vi "DataViewer.vi"() -> ()   [LabVIEW 2025]
uses:
  Controls/Dependand_Variables.ctl
  Controls/State.ctl
  <vilib>/Utility/miscctls.llb/LVRowAndColumnUnsignedTypeDef.ctl
panel:
  in  "Btt:Down":bool
  in  "Btt:Up":bool
  out "2D":T1
  out "Horizontal":T1
  out "Vertical":T1
  out "Duration [min]":dbl
  out "End":timestamp
  out "Begin":timestamp
  in  "Stop":bool
  out "Raw Data":i32(listbox)
  in  "Combo Box":string(combo)
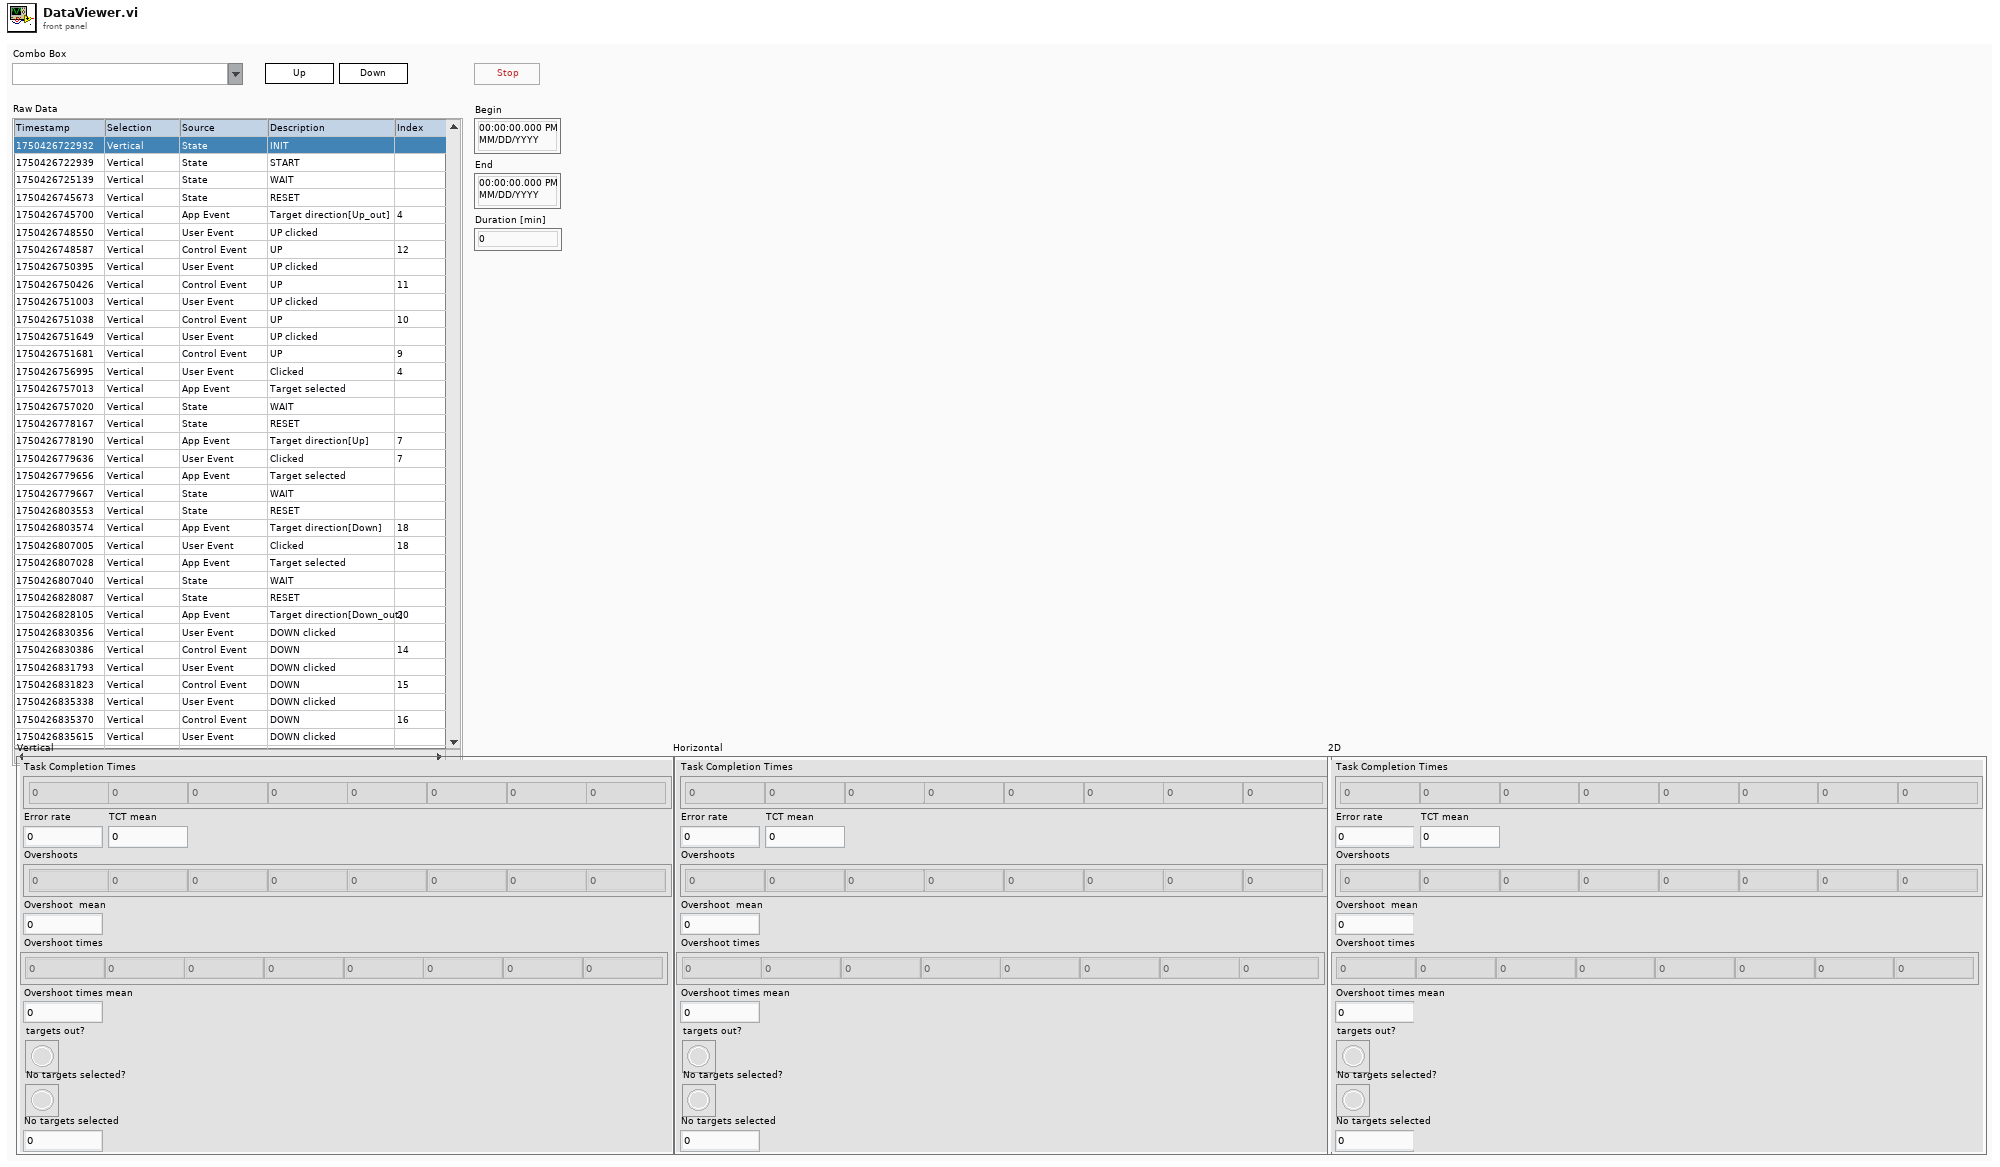
[diagram p1: front panel]
types:
  T1 = typedef "Dependand_Variables.ctl" = cluster{"Task Completion Times":dbl[], "TCT mean":dbl, "Error rate":i32, "Overshoots":i32[], "Overshoot  mean":dbl, "Overshoot times":dbl[], "Overshoot times mean":dbl, "targets out?":bool[], "No targets selected?":bool[], "No targets selected":i32}
  T2 = typedef "State.ctl" = enum16{"Init", "Idle", "Analyze", "End"}
  T3 = typedef "LVRowAndColumnUnsignedTypeDef.ctl" = cluster{"Row":u32, "Column":u32}
  T4 = typedef "LVComboBoxStrsAndValuesArrayTypeDef.ctl" = cluster{"String":string, "Value":string}[]
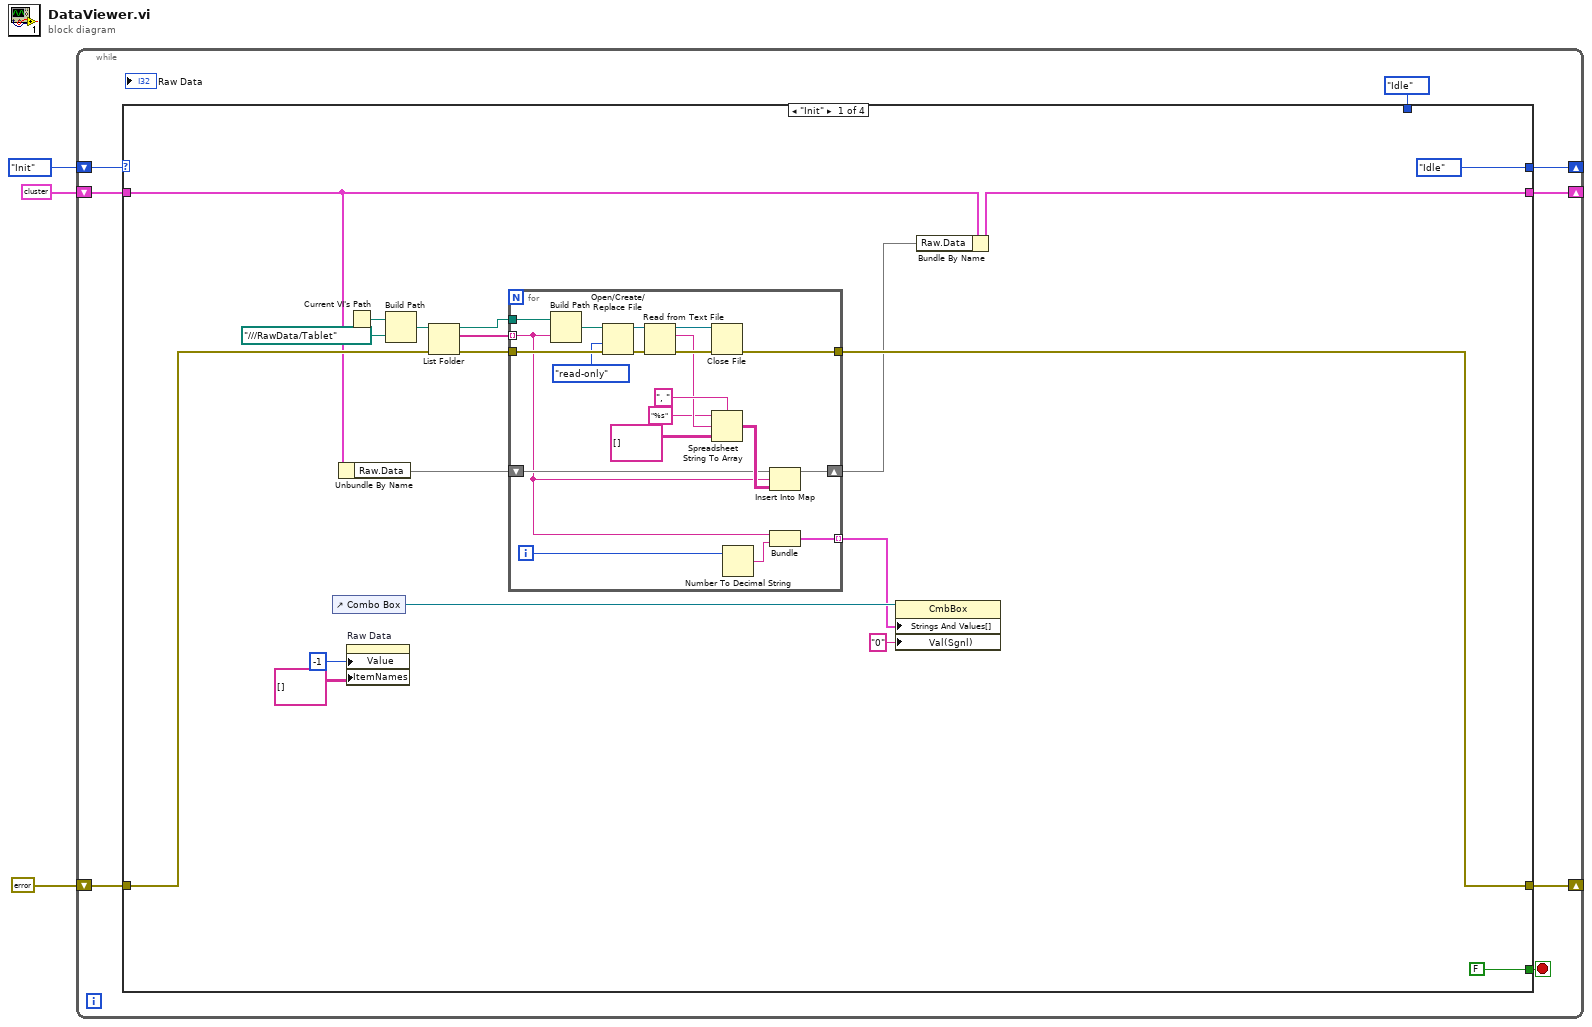
[diagram p0: block diagram]
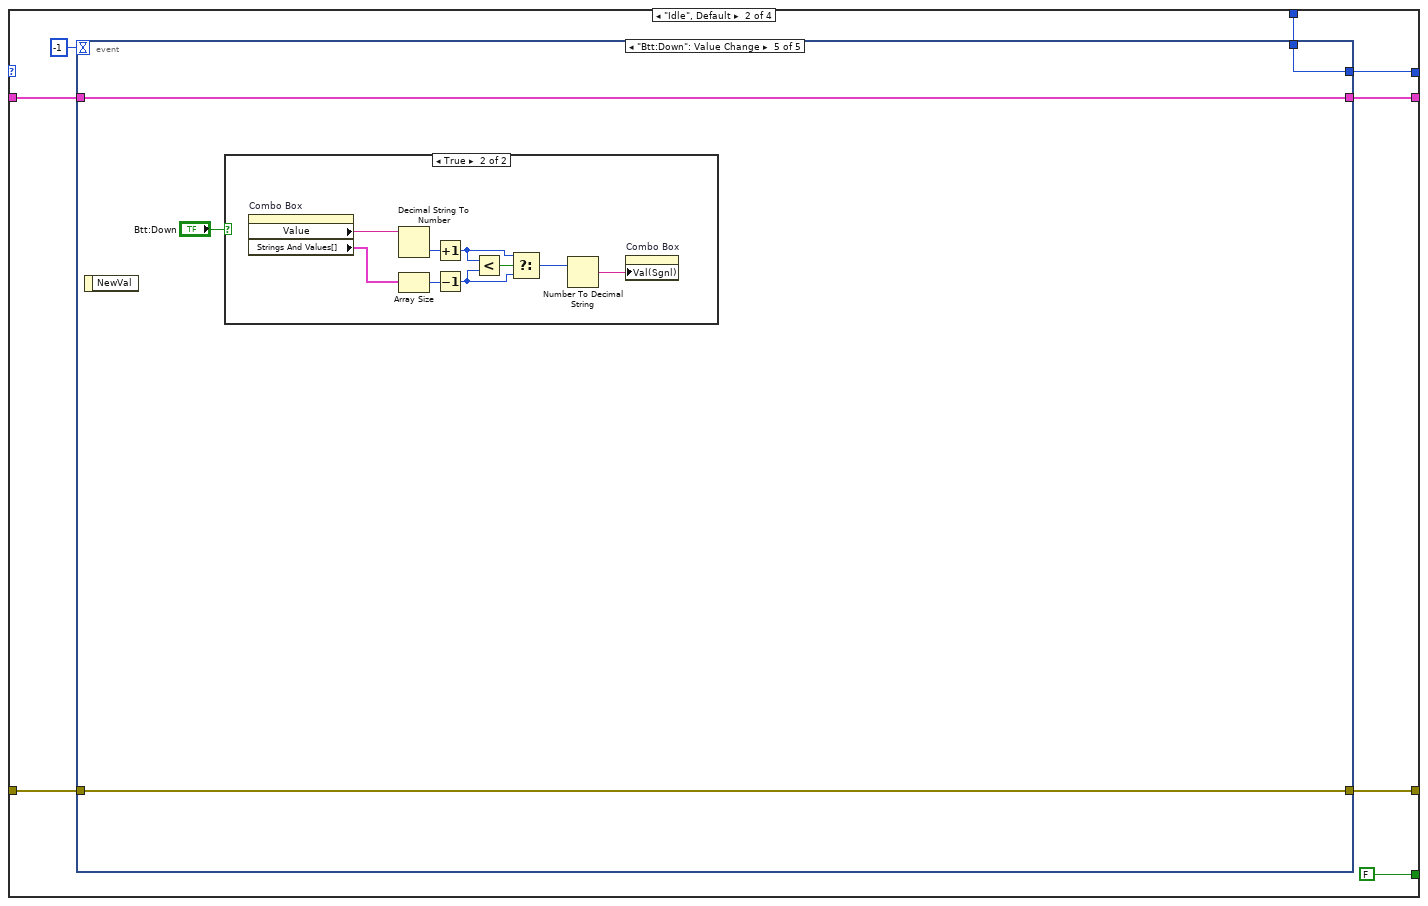
[diagram p2: hidden frame]
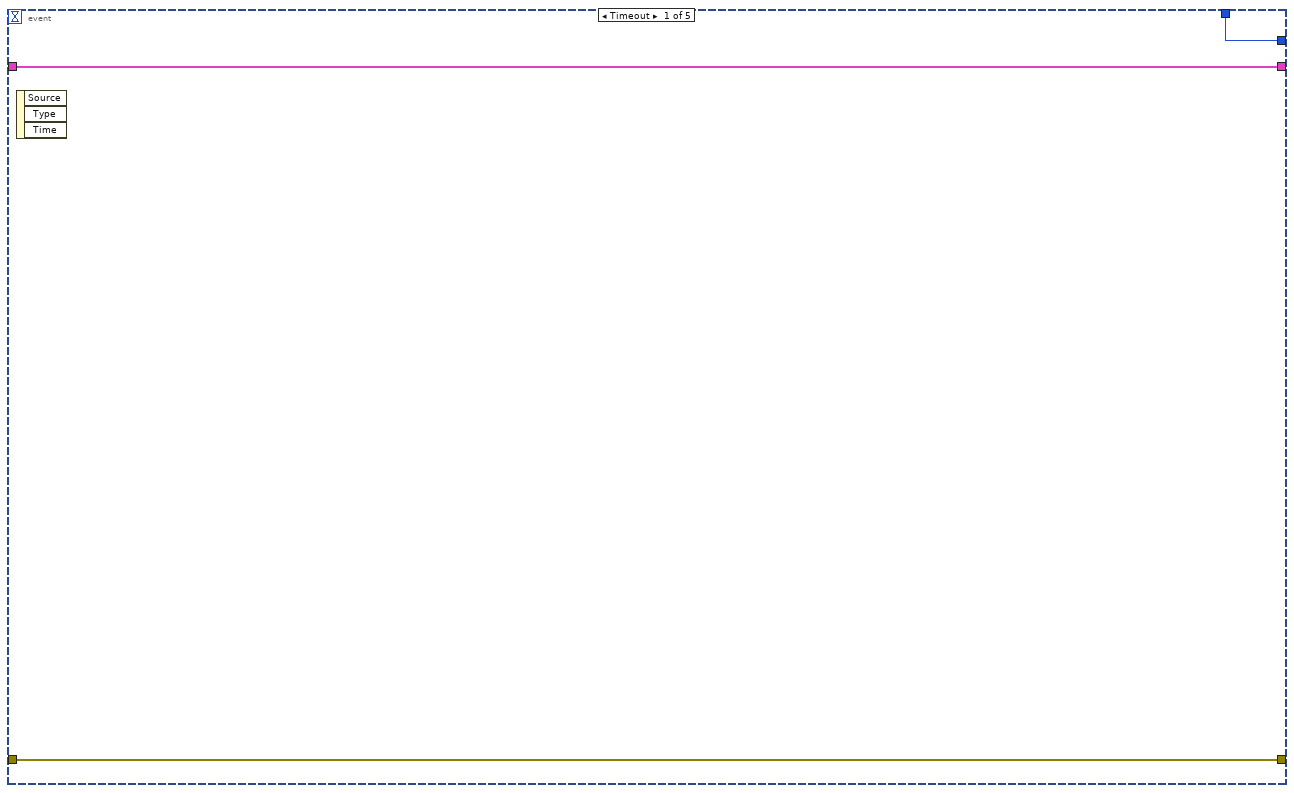
[diagram p3: hidden frame]
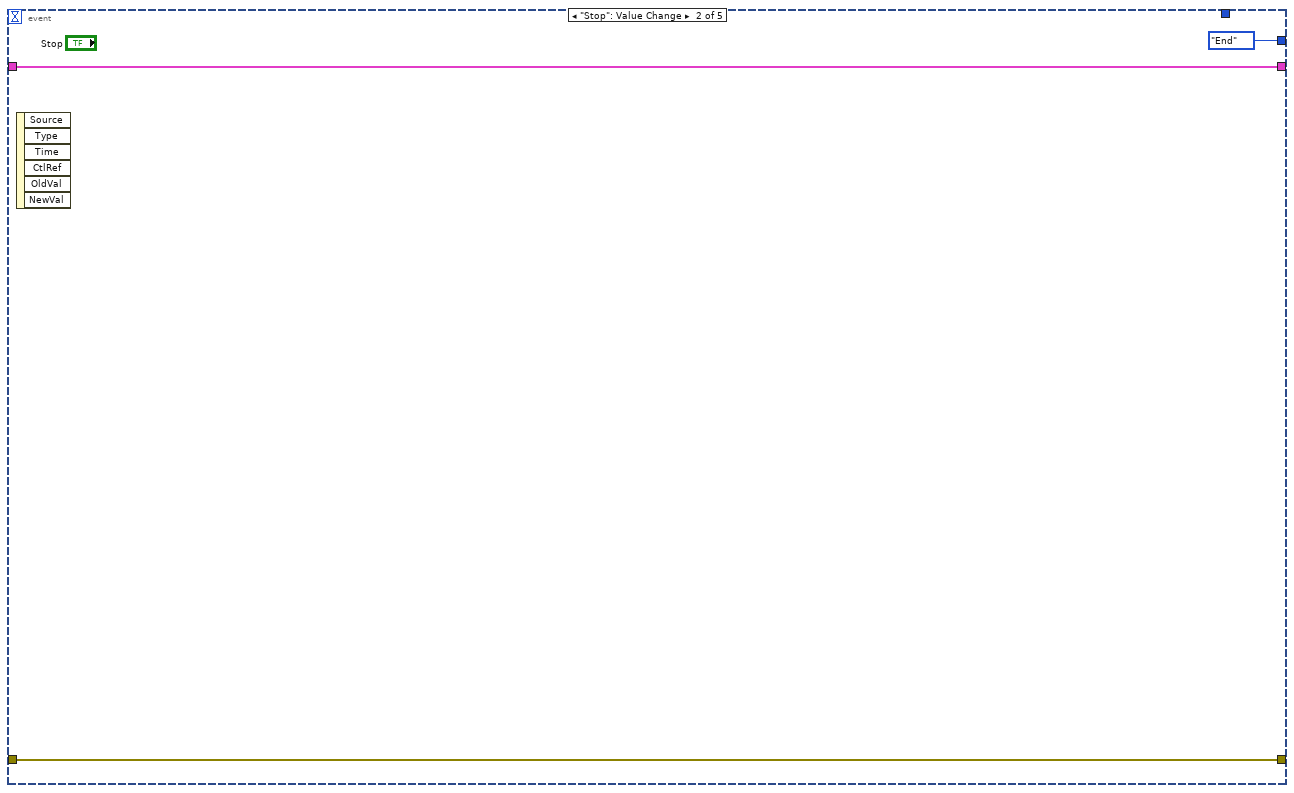
[diagram p4: hidden frame]
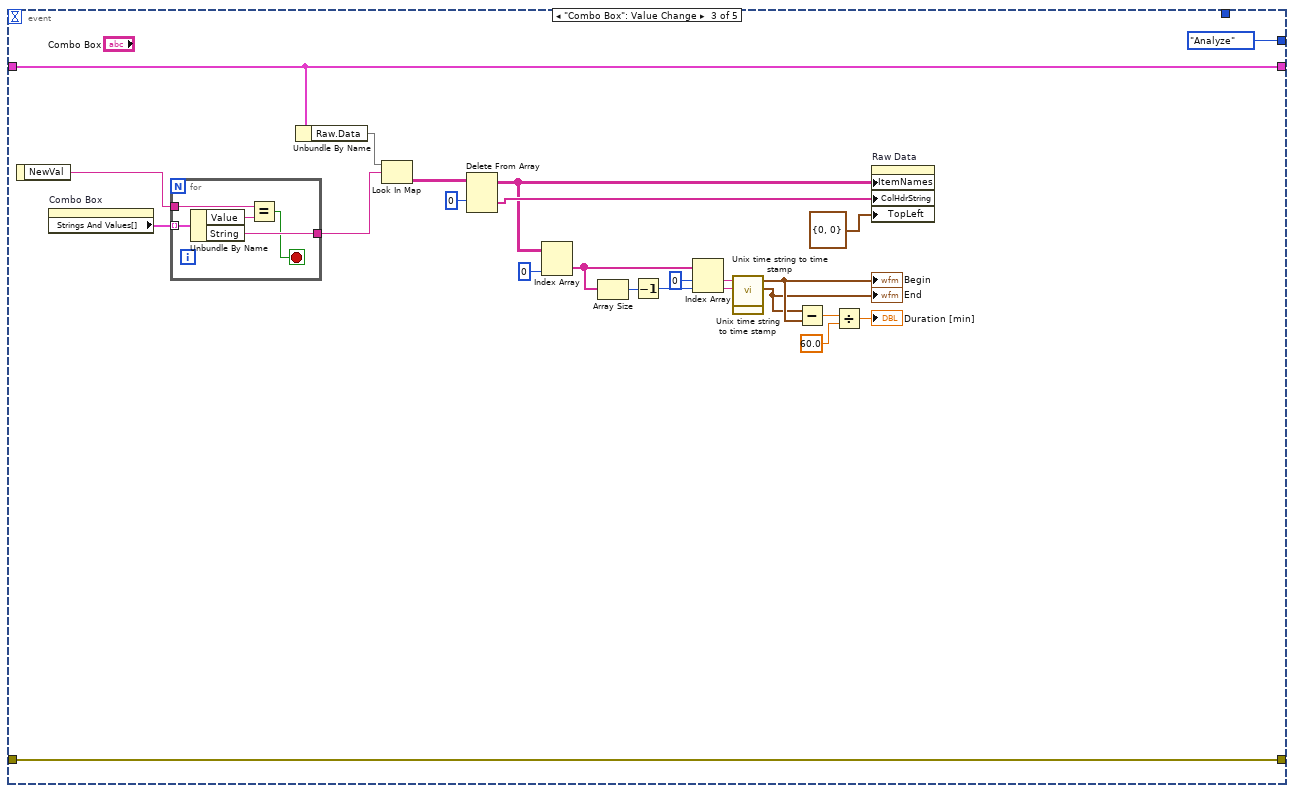
[diagram p5: hidden frame]
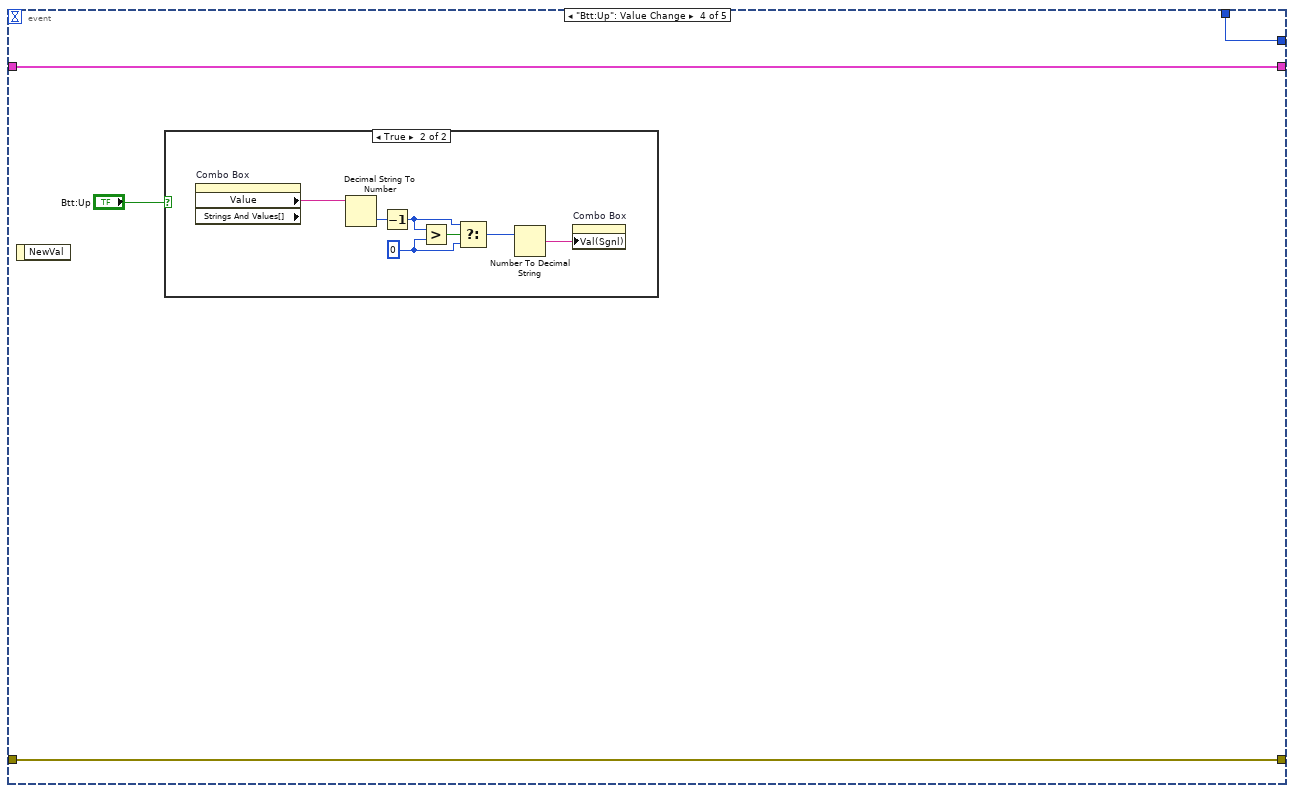
[diagram p6: hidden frame]
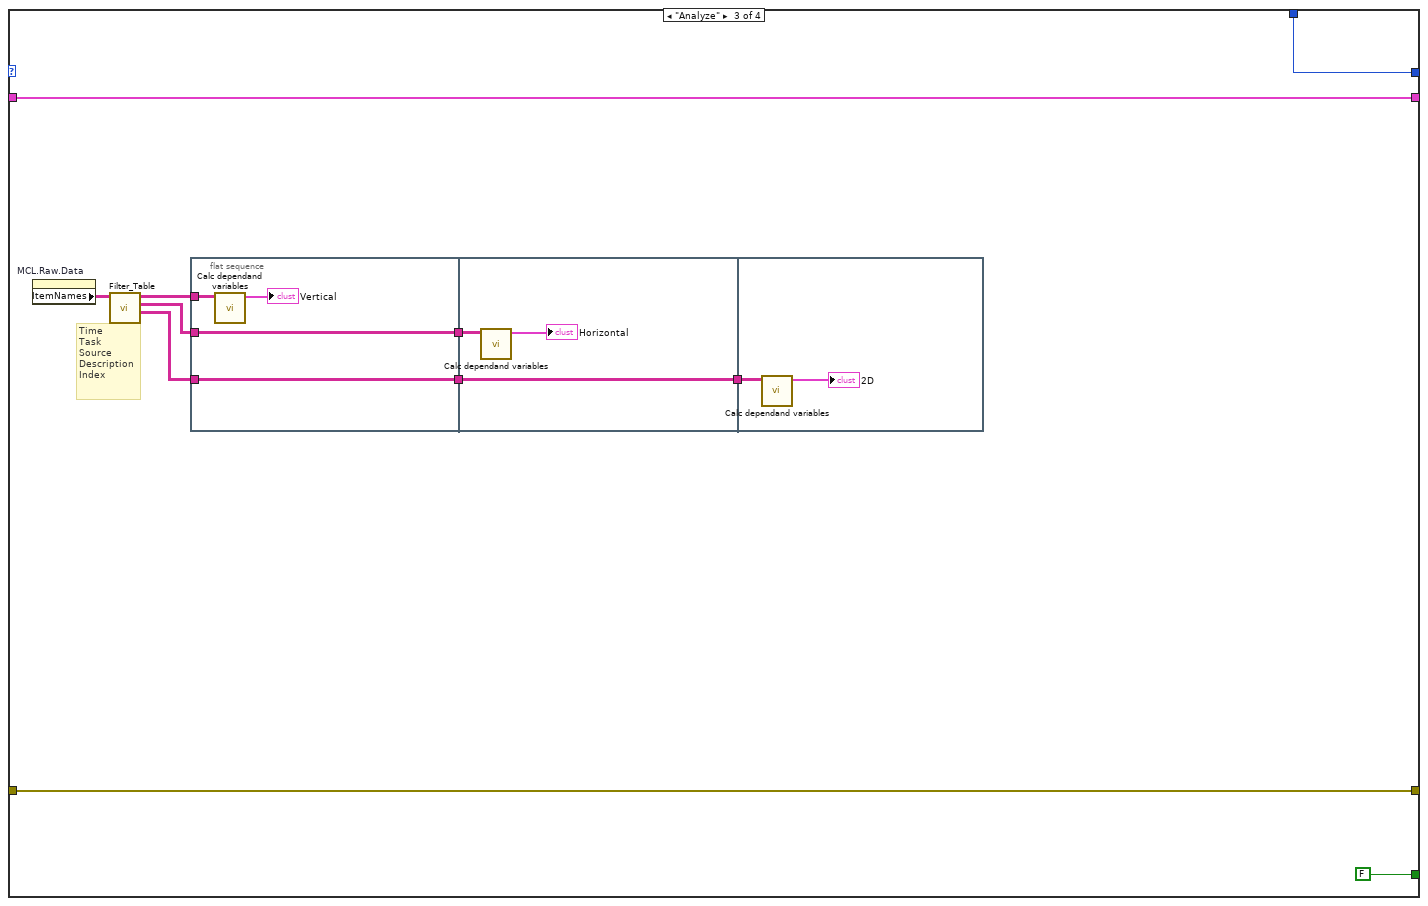
[diagram p9: hidden frame]
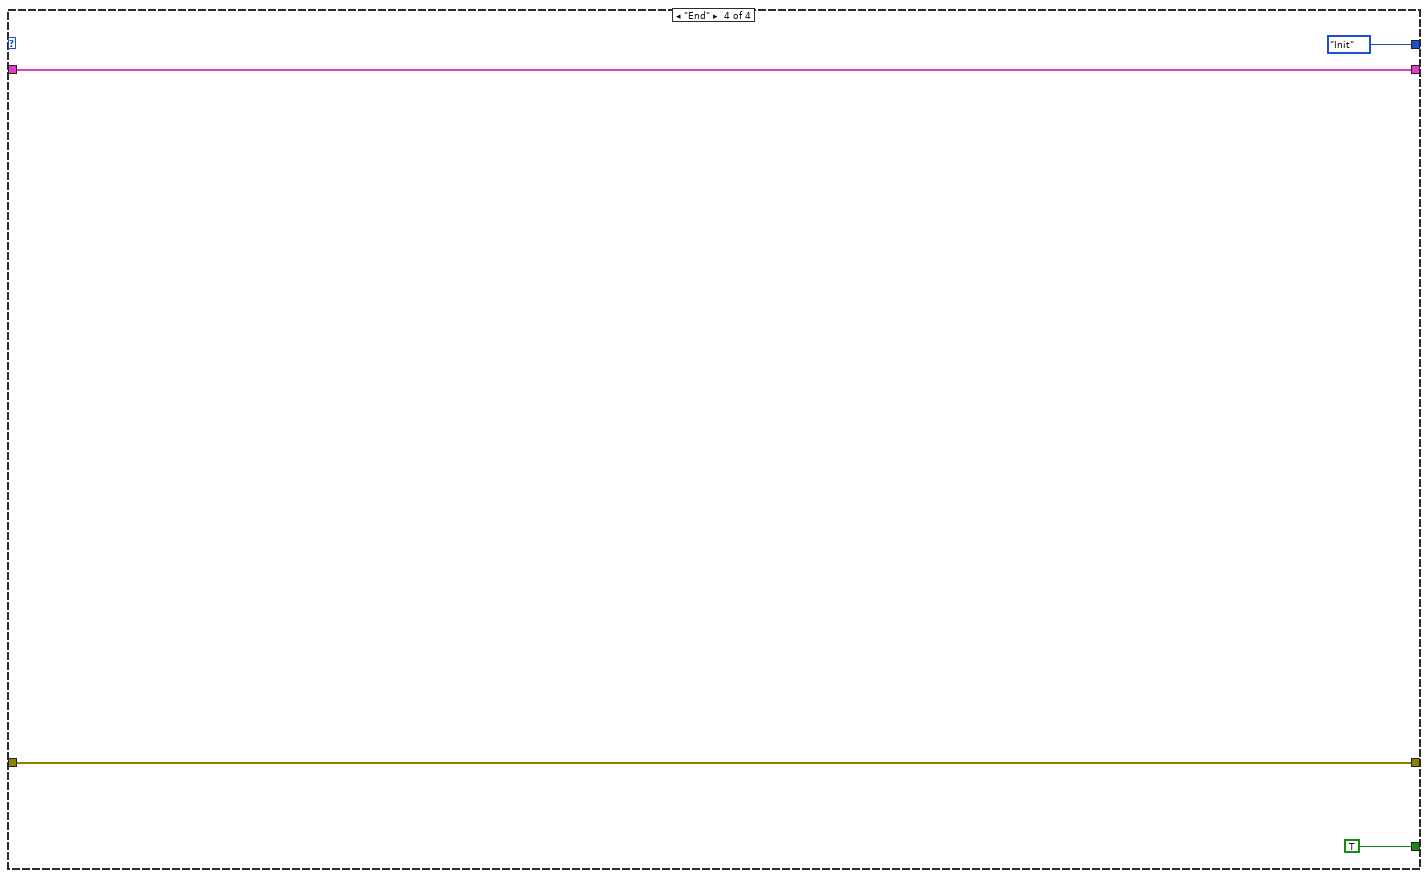
[diagram p10: hidden frame]
diagram:
  n1 = while {
    shift-right: [w9] -> _
    shift-left: errorcluster {"status"=FALSE, "code"=0, "source"=""} ("error constant") -> [w10]
    shift-right: [w8] -> _
    shift-left: State."Init" -> [w11]
    shift-right: [w5] -> _
    shift-left: cluster{"Raw.Data":map{string, string[][]}} {"Raw.Data"={}} -> [w6]
    stop <- w4 stop-if-true
    n2 = case shown="\"Init\"" w11 {
      tunnel: w10 -> [w26 w57 w126 w141]
      tunnel: [w25 w58 w126 w141] -> w9
      tunnel: [State."Idle" w55 w128 State."Init"] -> w8
      tunnel: State."Idle" -> [_ w54 w128 _]
      tunnel: w6 -> [w22 w52 w127 w138]
      tunnel: [w23 w53 w127 w138] -> w5
      tunnel: [FALSE FALSE FALSE TRUE] -> w4
      frame "Init" {
        n3 = control-ref of="Combo Box"() -> (w29:refnum<vi>)
        n4 = Unbundle By Name(w22) -> ("Raw.Data"=w21:map{string, string[][]})
        n5 = Current VI's Path() -> (path=w14:path)
        n6 = property on="Raw Data" class="MCListbox (strict)"("Value"=-1 ("Multicolumn Listbox"), "ItemNames"=string[][] [] ("Item Names")) -> ()  [unwired: 2 in, 2 out]
        n7 = Build Path(base path=w14, name or relative path=path "../../../RawData/Tablet") -> (appended path=w12:path)
        n8 = List Folder(path=w12, error in=w26) -> (path out=w28:path, filenames=w30:string[], error out=w27:errorcluster)  [unwired: 2 in, 1 out]
        n9 = for {
          tunnel: w27 -> [w50]
          tunnel: w28 -> [w45]
          tunnel: w30 -> [w32] mode=indexing
          tunnel: [w38] -> w25
          shift-right: [w35] -> w20
          shift-left: w21 -> [w36]
          tunnel: [w31] -> w16 mode=indexing
          i -> [w34]
          n10 = Build Path(base path=w45, name or relative path=w32) -> (appended path=w44:path)
          n11 = Open/Create/Replace File(file path (use dialog)=w44, error in=w50, access (0:read/write)=enum16{"read/write", "read-only", "write-only"}."read-only") -> (refnum out=w49:refnum<file>, error out=w48:errorcluster)  [unwired: 3 in, 1 out]
          n12 = Read from Text File(file (use dialog)=w49, error in=w48) -> (refnum out=w47:refnum<file>, text=w41:string, error out=w46:errorcluster)  [unwired: 2 in, 1 out]
          n13 = Close File(refnum=w47, error in=w46) -> (error out=w38:errorcluster)  [unwired: 1 out]
          n14 = Spreadsheet String To Array(delimiter (Tab)=", ", format string="%s", spreadsheet string=w41, array type (2D Dbl)=string[][] []) -> (array=w37:string[][])
          n15 = Number To Decimal String(number=w34) -> (decimal integer string=w33:string)  [unwired: 1 in]
          n16 = Insert Into Map(map in=w36, key=w32, value=w37) -> (map out=w35:map{string, string[][]})  [unwired: 2 out]
          n17 = Bundle(w32, w33) -> (w31:cluster{string, string})  [unwired: 1 in]
        }
        n18 = property class="CmbBox"(reference=w29, "Strings And Values[]"=w16, "Val(Sgnl)"="0" ("Value (Signaling)")) -> ()  [unwired: 1 in, 2 out]
        n19 = Bundle By Name(cluster=w22, "Raw.Data"=w20) -> (w23:cluster{"Raw.Data":map{string, string[][]}})
      }
      frame "Idle", Default {
        n20 = event shown="[4] \"Btt:Down\": Value Change" {
          selector: _ -> [_ _ _ _ _]
          dyn-events: _ -> [_ _ _ _ _]
          timeout: -1 -> [_ _ _ _ _]
          tunnel: [w61 w64 w69 w95 w106] -> w58
          tunnel: w57 -> [w61 w64 w69 w95 w106]
          tunnel: [w60 State."End" State."Analyze" w97 w108] -> w55
          tunnel: w54 -> [w60 _ _ w97 w108]
          tunnel: [w59 w62 w88 w96 w107] -> w53
          tunnel: w52 -> [w59 w62 w88 w96 w107]
          event Timeout {
            n21 = event-data() -> ()  [unwired: 1 in, 3 out]
          }
          event "Stop": Value Change {
            n22 = event-data() -> ()  [unwired: 1 in, 6 out]
          }
          event "Combo Box": Value Change {
            n23 = event-data() -> ("NewVal"=w66:string)  [unwired: 1 in]
            n24 = property on="Combo Box" class="CmbBox"() -> ("Strings And Values[]"=w67:T4)  [unwired: 2 in, 2 out]
            n25 = for {
              tunnel: w67 -> [w93] mode=indexing
              tunnel: w66 -> [w91]
              tunnel: [w90] -> w65
              stop <- w89 stop-if-true
              n26 = Unbundle By Name(w93) -> ("Value"=w92:string, "String"=w90:string)
              n27 = Equal?(x=w91, y=w92) -> (x = y?=w89:bool)
            }
            n28 = Unbundle By Name(w88) -> ("Raw.Data"=w87:map{string, string[][]})
            n29 = Look In Map(map=w87, key=w65) -> (value=w86:string[][])  [unwired: 1 in, 1 out]
            n30 = Delete From Array(array=w86, index (row)=0) -> (deleted portion=w84:string[], array with subset deleted=w82:string[][])  [unwired: 2 in]
            n31 = Index Array(array=w82, index (col)=0 ("disabled index (col)")) -> (element=w80:string[])  [unwired: 1 in]
            n32 = Array Size(array=w80) -> (size(s)=w79:i32)
            n33 = Decrement(x=w79) -> (x-1=w78:i32)
            n34 = Index Array(array=w80, index #1=0 ("index"), index #2=w78) -> (element #1=w73:string, element #2=w72:string)
            n35 = call "Unix time string to time stamp.vi"("Unix time string [ms]"=w73) -> ("Time stamp"=w71:timestamp)  [unwired: 4 in]
            "Begin" <- w71
            n36 = call "Unix time string to time stamp.vi"("Unix time string [ms]"=w72) -> ("Time stamp"=w70:timestamp)  [unwired: 4 in]
            "End" <- w70
            n37 = Subtract(x=w70, y=w71) -> (x-y=w77:dbl)
            n38 = Divide(x=w77, y=60.0) -> (x/y=→"Duration [min]":dbl)
            n39 = property on="Raw Data" class="MCListbox (strict)"("ItemNames"=w82, "ColHdrString"=w84, "TopLeft"=T3 {"Row"=0, "Column"=0} ("Top Left Visible Cell")) -> ()  [unwired: 2 in, 2 out]
          }
          event "Btt:Up": Value Change {
            n40 = event-data() -> ()  [unwired: 1 in, 1 out]
            n41 = case shown="True" "Btt:Up" {
              frame False {
              }
              frame True {
                w98 = 0 ("y")
                n42 = property on="Combo Box" class="CmbBox" props=["Value", "Strings And Values[]"]() -> ("Value"=w104:string)  [unwired: 2 in, 3 out]
                n43 = Decimal String To Number(string=w104) -> (number=w103:i32)  [unwired: 2 in, 1 out]
                n44 = Decrement(x=w103) -> (x-1=w100:i32)
                n45 = Greater?(x=w100, y=w98) -> (0:w101:bool)
                n46 = Select(t=w100, s=w101, f=w98) -> (s? t:f=w99:i32)
                n47 = Number To Decimal String(number=w99) -> (decimal integer string=w102:string)  [unwired: 1 in]
                n48 = property on="Combo Box" class="CmbBox"("Val(Sgnl)"=w102) -> ()  [unwired: 2 in, 2 out]
              }
            }
          }
          event "Btt:Down": Value Change {
            n49 = event-data() -> ()  [unwired: 1 in, 1 out]
            n50 = case shown="True" "Btt:Down" {
              frame False {
              }
              frame True {
                n51 = property on="Combo Box" class="CmbBox"() -> ("Value"=w117:string, "Strings And Values[]"=w114:T4)  [unwired: 2 in, 2 out]
                n52 = Decimal String To Number(string=w117) -> (number=w116:i32)  [unwired: 2 in, 1 out]
                n53 = Array Size(array=w114) -> (size(s)=w113:i32)
                n54 = Increment(x=w116) -> (x+1=w111:i32)
                n55 = Decrement(x=w113) -> (x-1=w110:i32)
                n56 = Less?(x=w111, y=w110) -> (x < y?=w112:bool)
                n57 = Select(t=w111, s=w112, f=w110) -> (s? t:f=w109:i32)
                n58 = Number To Decimal String(number=w109) -> (decimal integer string=w115:string)  [unwired: 1 in]
                n59 = property on="Combo Box" class="CmbBox"("Val(Sgnl)"=w115) -> ()  [unwired: 2 in, 2 out]
              }
            }
          }
        }
      }
      frame "Analyze" {
        # "Time\nTask\nSource\nDescription\nIndex"
        n60 = property on="MCL.Raw.Data" class="MCListbox (strict)"() -> ("ItemNames"=w125:string[][])  [unwired: 2 in, 2 out]
        n61 = call "Filter_Table.vi"("Table in"=w125) -> ("2D"=w119:string[][], "Horizontal"=w122:string[][], "Vertical"=w124:string[][])  [unwired: 8 in]
        n62 = flat-sequence {
          tunnel: w124 -> [w132]
          tunnel: w122 -> [w131]
          tunnel: [w131] -> w121
          tunnel: w119 -> [w130]
          tunnel: [w130] -> w118
          tunnel: w121 -> [w135]
          tunnel: [w134] -> w120
          tunnel: w118 -> [w134]
          tunnel: w120 -> [w137]
          frame #0 {
            n63 = call "Calc dependand variables.vi"("Item Names"=w132) -> ("Dependand Variables"=→"Vertical":T1)  [unwired: 10 in]
          }
          frame #1 {
            n64 = call "Calc dependand variables.vi"("Item Names"=w135) -> ("Dependand Variables"=→"Horizontal":T1)  [unwired: 10 in]
          }
          frame #2 {
            n65 = call "Calc dependand variables.vi"("Item Names"=w137) -> ("Dependand Variables"=→"2D":T1)  [unwired: 10 in]
          }
        }
      }
      frame "End" {
      }
    }
  }
